vi "In S.vi"(9 "VISA resource name 2":refnum<visa-resource-name>="com4", 10 "设定温度":string) -> ()   [LabVIEW 2021]
uses:
  <vilib>/Instr/_visa.llb/VISA Configure Serial Port (Instr).vi
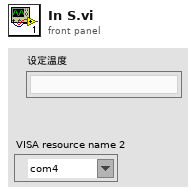
[diagram p1: front panel]
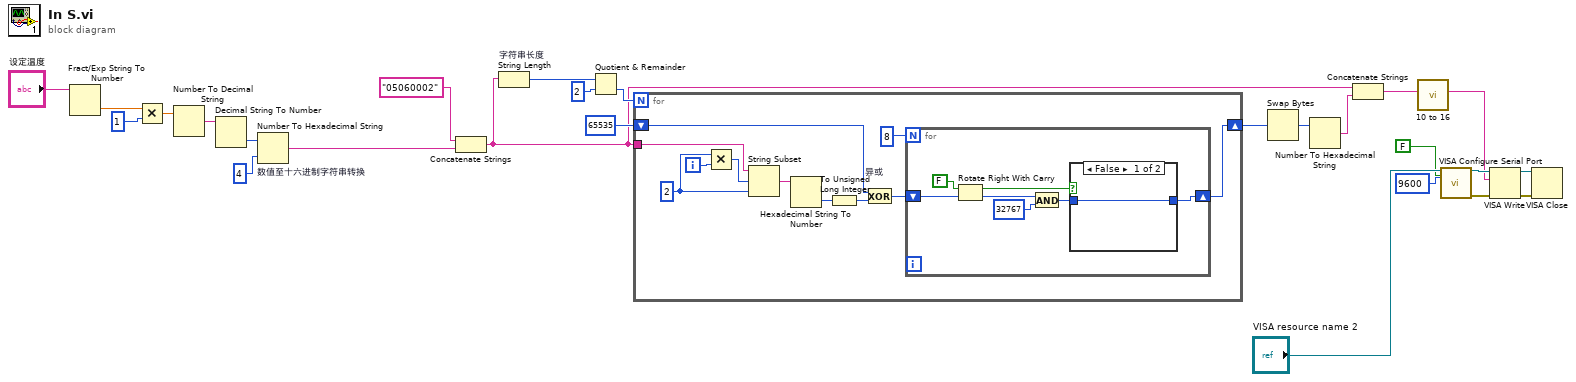
[diagram p0: block diagram]
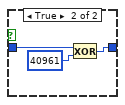
[diagram p2: hidden frame]
diagram:
  n1 = Fract/Exp String To Number(string="设定温度") -> (number=w13:dbl)  [unwired: 3 in, 1 out]
  n2 = Multiply(x=w13, y=1) -> (x*y=w12:dbl)
  n3 = Number To Decimal String(number=w12) -> (decimal integer string=w9:string)  [unwired: 1 in]
  n4 = Decimal String To Number(string=w9) -> (number=w23:i32)  [unwired: 2 in, 1 out]
  n5 = Number To Hexadecimal String "数值至十六进制字符串转换"(1:4, 2:w23) -> (0:w24:string)
  n6 = Concatenate Strings("05060002" ("写入缓冲区"), w24) -> (w15:string)
  n7 = String Length "字符串长度"(string=w15) -> (length=w20:i32)
  n8 = Quotient & Remainder(x=w20, y=2) -> (floor(x/y)=w22:i32)  [unwired: 1 out]
  n9 = for {
    N: w22 -> [_]
    tunnel: w15 -> [w37]
    shift-right: [w27] -> w18
    shift-left: 65535 -> [w28]
    i -> [w35]
    w36 = 2
    n10 = Multiply(x=w36, y=w35) -> (x*y=w34:i32)
    n11 = String Subset ("截取字符串")(string=w37, offset (0)=w34, length (rest)=w36) -> (substring=w33:string)
    n12 = Hexadecimal String To Number ("十六进制数字符串至数值转换")(string=w33) -> (number=w32:u32)  [unwired: 2 in, 1 out]
    n13 = To Unsigned Long Integer ("转换为无符号长整型")(number=w32) -> (unsigned 32bit integer=w31:u32)
    n14 = Exclusive Or "异或"(1:w31, 2:w28) -> (0:w29:u32)
    n15 = for {
      N: 8 -> [_]
      shift-right: [w42] -> w27
      shift-left: w29 -> [w44]
      n16 = Rotate Right With Carry(2:w44, 3:FALSE) -> (0:w40:u32, 1:w41:bool)
      n17 = And(x=w40, y=u32 32767) -> (x .and. y?=w39:u32)
      n18 = case shown="False" w41 {
        tunnel: w39 -> [w45 w47]
        tunnel: [w45 w46] -> w42
        frame False {
        }
        frame True {
          n19 = Exclusive Or(1:u32 40961, 2:w47) -> (0:w46:u32)
        }
      }
    }
  }
  n20 = Swap Bytes ("交换字节")(anything=w18) -> (byte swapped=w17:u32)
  n21 = Number To Hexadecimal String ("数值至十六进制字符串转换")(2:w17) -> (0:w16:string)  [unwired: 1 in]
  n22 = Concatenate Strings(w15, w16) -> (w14:string)
  n23 = call "10 to 16.vi"("字符串"=w14) -> ("字符串 2"=w3:string)  [unwired: 10 in]
  n24 = call-poly "VISA Configure Serial Port"("VISA resource name"="VISA resource name 2", "Enable Termination\nChar (T)"=FALSE ("确定按钮"), "baud rate (9600)"=u32 9600) -> ("VISA resource name out"=w7:refnum<visa-resource-name>, "error out"=w4:errorcluster)  [unwired: 11 in]
  n25 = VISA Write ("VISA写入")(VISA resource name=w7, write buffer=w3, error in (no error)=w4) -> (VISA resource name out=w6:refnum<visa-resource-name>, error out=w5:errorcluster)  [unwired: 1 out]
  n26 = VISA Close(VISA resource name=w6, error in (no error)=w5) -> ()  [unwired: 1 out]
